vi "Create_Temporary_Path_forSWF_embedded_into_HTML.vi"(7 "offset past match":i32, 8 "error in (no error)":errorcluster, 9 "Identifying_String":string="img src=\"", 10 "FolderName":string, 11 "Dencrypted text":string) -> (0 "error out":errorcluster, 1 "fileName":string, 2 "Temp_PATH":path, 3 "HTML_wPathChanged":string, 5 "offset past match":i32)   [LabVIEW 2016]
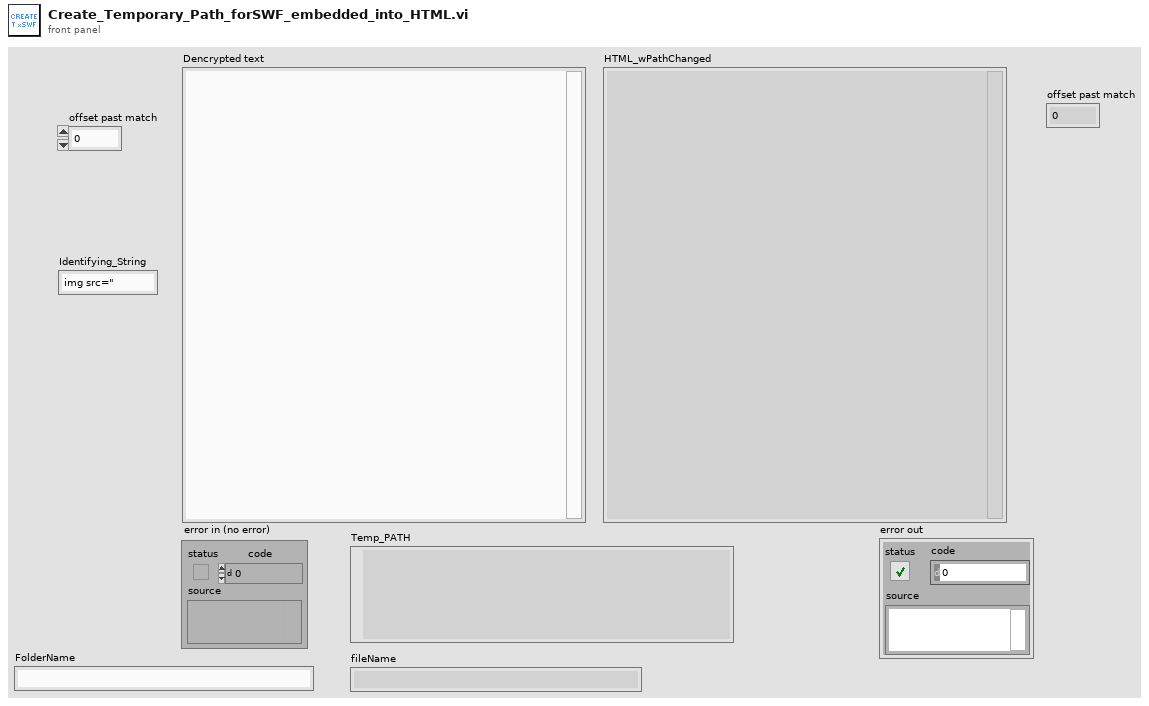
[diagram p1: front panel]
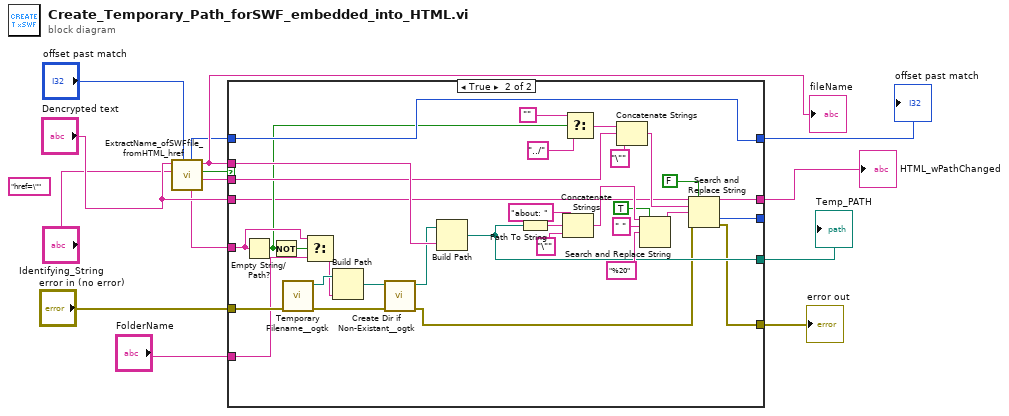
[diagram p0: block diagram]
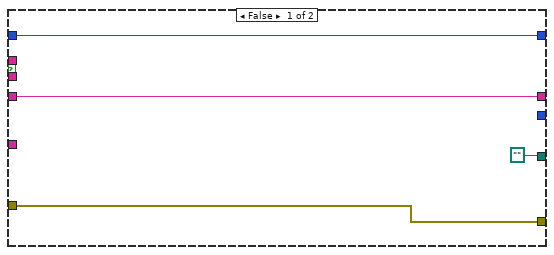
[diagram p2: hidden frame]
diagram:
  (unwired) "href=\"" ("Identifying_String")
  n1 = call "ExtractName_ofSWFfile_fromHTML_href.vi"("offset in"="offset past match", "Identifying_String"="Identifying_String", "Dencrypted HTML"="Dencrypted text") -> ("AllText"=w7:string, "Found?"=w6:bool, "fileName"=w14:string, "FolderName"=w2:string, "offset past match"=w5:i32)  [unwired: 3 in, 1 out]
  "fileName" <- w14
  n2 = case shown="True" w6 {
    tunnel: w14 -> [_ w51]
    tunnel: "Dencrypted text" -> [w15 w25]
    tunnel: "error in (no error)" -> [w18 w49]
    tunnel: [w15 w20] -> w11
    tunnel: [w18 w22] -> w10
    tunnel: [path "" w24] -> w9
    tunnel: w7 -> [_ w28]
    tunnel: [w17 w46] -> w4
    tunnel: w5 -> [w17 w46]
    tunnel: w2 -> [_ w43]
    tunnel: "FolderName" -> [_ w41]
    tunnel: [_ w21] -> _
    frame False {
    }
    frame True {
      n3 = Empty String/Path?(string/path=w43) -> (empty?=w26:bool)
      n4 = Not(x=w26) -> (.not. x?=w44:bool)
      n5 = call <userlib>:"Temporary Filename__ogtk.vi"("error in (no error)"=w49) -> ("error out"=w48:errorcluster, "file in tmp dir"=w50:path)  [unwired: 5 in]
      n6 = Select(t=w43, s=w44, f=w41) -> (s? t:f=w42:string)
      n7 = Build Path(base path=w50, name or relative path=w42) -> (appended path=w47:path)
      n8 = call <userlib>:"Create Dir if Non-Existant__ogtk.vi"("error in (no error)"=w48, "Directory Path"=w47) -> ("error out"=w23:errorcluster, "dup Directory Path"=w45:path)  [unwired: 7 in, 1 out]
      n9 = Build Path(base path=w45, name or relative path=w51) -> (appended path=w24:path)
      n10 = Path To String(path=w24) -> (string=w36:string)
      n11 = Concatenate Strings("about: " ("string"), w36, "\"") -> (w33:string)
      n12 = Select(t="", s=w26, f="../" ("search string")) -> (s? t:f=w35:string)
      n13 = Concatenate Strings(w35, w28, "\"") -> (w37:string)
      n14 = Search and Replace String(replace all?=TRUE ("replace all? (F)"), input string=w33, search string=" ", replace string="%20" ("replace string (\"\")")) -> (result string=w32:string)  [unwired: 4 in, 3 out]
      n15 = Search and Replace String(replace all?=FALSE ("replace all? (F)"), input string=w25, search string=w37, replace string=w32, error in=w23) -> (result string=w20:string, offset past replacement=w21:i32, error out=w22:errorcluster)  [unwired: 3 in, 1 out]
    }
  }
  "HTML_wPathChanged" <- w11
  "error out" <- w10
  "Temp_PATH" <- w9
  "offset past match" <- w4
